vi "Untitled 1.vi"   [LabVIEW 2016]
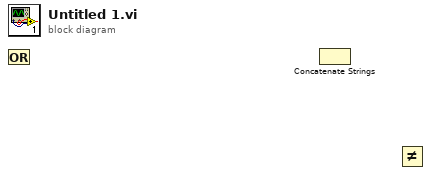
[diagram p0: block diagram]
diagram:
  n1 = Or() -> ()  [unwired: 2 in, 1 out]
  n2 = Concatenate Strings() -> ()  [unwired: 2 in, 1 out]
  n3 = Not Equal?() -> ()  [unwired: 2 in, 1 out]
